vi "niFPGA BW CU Order 2 (16-bit).vi"(0 "filter state in":T1, 1 "reset":bool, 5 "input data":i16, 7 "accumulator in":i32, 9 "adder in":i32, 11 "iteration":u8, 12 "in shift":i8=-1, 13 "lowpass?":bool) -> (4 "filter state out":T1, 6 "state to multiply":i32, 8 "accumulator out":i32, 10 "adder out":i32, 15 "terminate":bool)   [LabVIEW 2017]
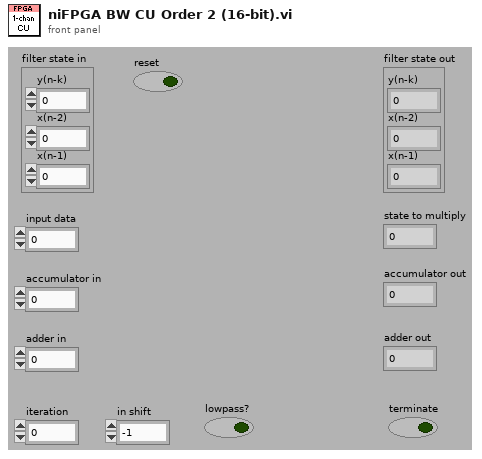
[diagram p1: front panel]
types:
  T1 = cluster{"y(n-k)":i32, "x(n-2)":i16, "x(n-1)":i16}
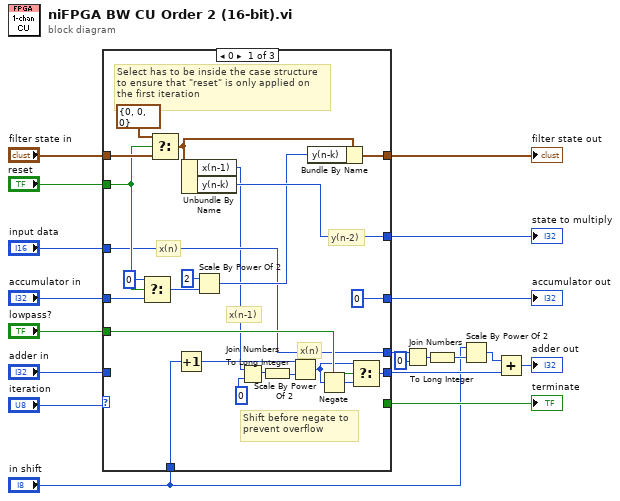
[diagram p0: block diagram]
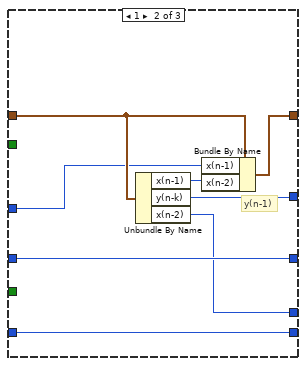
[diagram p2: hidden frame]
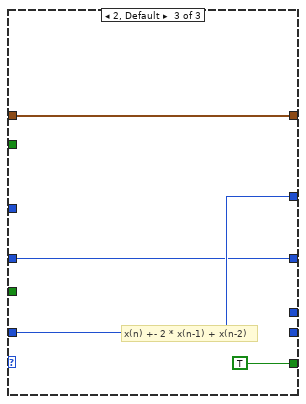
[diagram p3: hidden frame]
diagram:
  n1 = case shown="0" "iteration" {
    tunnel: [w42 w44 w51] -> w10
    tunnel: "input data" -> [w24 w43 _]
    tunnel: [w22 w50 _] -> w7
    tunnel: "adder in" -> [_ w50 w54]
    tunnel: [w37 w49 w54] -> w9
    tunnel: [w24 w47 _] -> w6
    tunnel: [0 ("Numeric") w48 w52] -> w8
    tunnel: [_ _ TRUE] -> w5
    tunnel: "reset" -> [w29 _ _]
    tunnel: "accumulator in" -> [w31 w48 w52]
    tunnel: "filter state in" -> [w30 w45 w51]
    tunnel: "in shift" -> [w28 _ _]
    tunnel: "lowpass?" -> [w25 _ _]
    frame 0 {
      # "Shift before negate to\nprevent overflow"
      # "Select has to be inside the case structure\nto ensure that \"reset\" is only applied on\nthe first iteration"
      # "x(n)"
      # "x(n)"
      # "x(n-1)"
      # "y(n-2)"
      n2 = Select(t=0, s=w29, f=w31) -> (s? t:f=w32:i32)
      n3 = Select(t=T1 {"y(n-k)"=0, "x(n-2)"=0, "x(n-1)"=0} ("output cluster"), s=w29, f=w30) -> (s? t:f=w34:T1)
      n4 = Increment(x=w28) -> (x+1=w27:i8)
      n5 = Unbundle By Name(w34) -> ("x(n-1)"=w23:i16, "y(n-k)"=w37:i32)
      n6 = Scale By Power Of 2(n=2, x=w32) -> (x*2^n=w36:i32)
      n7 = Join Numbers(hi=w23, lo=i16 0) -> ((hi.lo)=w41:u32)
      n8 = To Long Integer(number=w41) -> (32bit integer=w21:i32)
      n9 = Scale By Power Of 2(n=w27, x=w21) -> (x*2^n=w20:i32)
      n10 = Bundle By Name(cluster=w34, "y(n-k)"=w36) -> (w42:T1)
      n11 = Negate(x=w20) -> (-x=w26:i32)
      n12 = Select(t=w20, s=w25, f=w26) -> (s? t:f=w22:i32)
    }
    frame 1 {
      # "y(n-1)"
      n13 = Unbundle By Name(w45) -> ("x(n-1)"=w46:i16, "y(n-k)"=w49:i32, "x(n-2)"=w47:i16)
      n14 = Bundle By Name(cluster=w45, "x(n-1)"=w43, "x(n-2)"=w46) -> (w44:T1)
    }
    frame 2, Default {
      # "x(n) +- 2 * x(n-1) + x(n-2)"
    }
  }
  "filter state out" <- w10
  "state to multiply" <- w9
  "terminate" <- w5
  "accumulator out" <- w8
  n15 = Join Numbers(hi=w6, lo=i16 0) -> ((hi.lo)=w18:u32)
  n16 = To Long Integer(number=w18) -> (32bit integer=w17:i32)
  n17 = Scale By Power Of 2(n="in shift", x=w17) -> (x*2^n=w19:i32)
  n18 = Add(x=w19, y=w7) -> (x+y=→"adder out":i32)
